vi "Puntero_al_indice.vi"(10 "Numeric in":i32, 11 "N in":dbl) -> (2 "N out":dbl, 3 "Numeric out":i32)   [LabVIEW 2016]
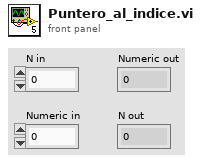
[diagram p1: front panel]
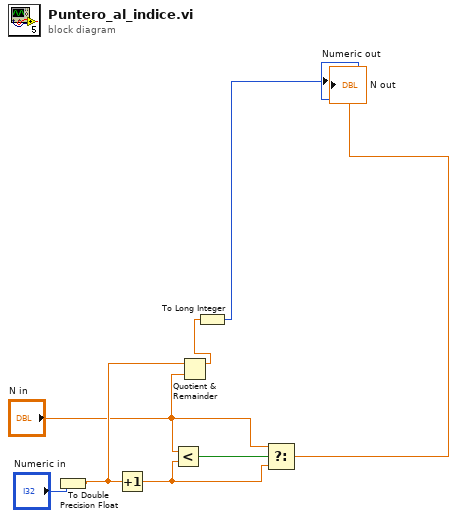
[diagram p0: block diagram]
diagram:
  n1 = To Double Precision Float(number="Numeric in") -> (double precision float=w5:dbl)
  n2 = Increment(x=w5) -> (x+1=w4:dbl)
  n3 = Less?(x="N in", y=w4) -> (x < y?=w2:bool)
  n4 = Quotient & Remainder(x=w5, y="N in") -> (x-y*floor(x/y)=w6:dbl)  [unwired: 1 out]
  n5 = To Long Integer(number=w6) -> (32bit integer=→"Numeric out":i32)
  n6 = Select(t="N in", s=w2, f=w4) -> (s? t:f=→"N out":dbl)
